vi "Errors to Item Names.vi"(5 "scope":T1, 7 "error list <top>":variant, 8 "error in (no error)":errorcluster, 11 "displayed errors in":T2[](array[typedef])) -> (0 "error out":errorcluster, 2 "item names":string[][](array[string]), 3 "displayed errors out":T2[](array[typedef]))   [LabVIEW 2017]
uses:
  Error List/Error Owner and ID.ctl
  Error List/Scope.ctl
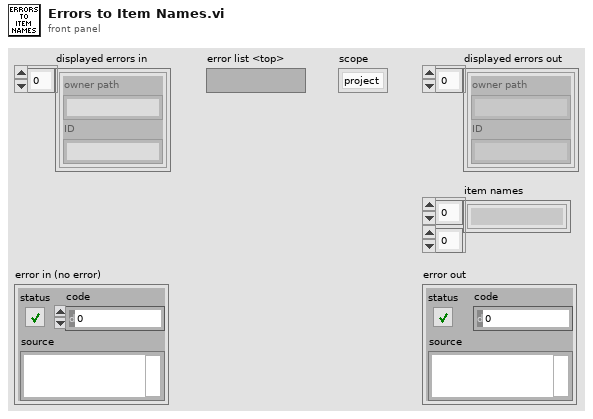
[diagram p1: front panel]
types:
  T1 = typedef "Scope.ctl" = enum16{"project", "global"}
  T2 = typedef "Error Owner and ID.ctl" = cluster{"owner path":string, "ID":string}
  T3 = typedef "Error Owners and IDs.ctl" = cluster{"owner path":string, "error IDs":string[]}
  T4 = typedef "Error File Management.lvlib/NI Error.ctl" = errorcluster
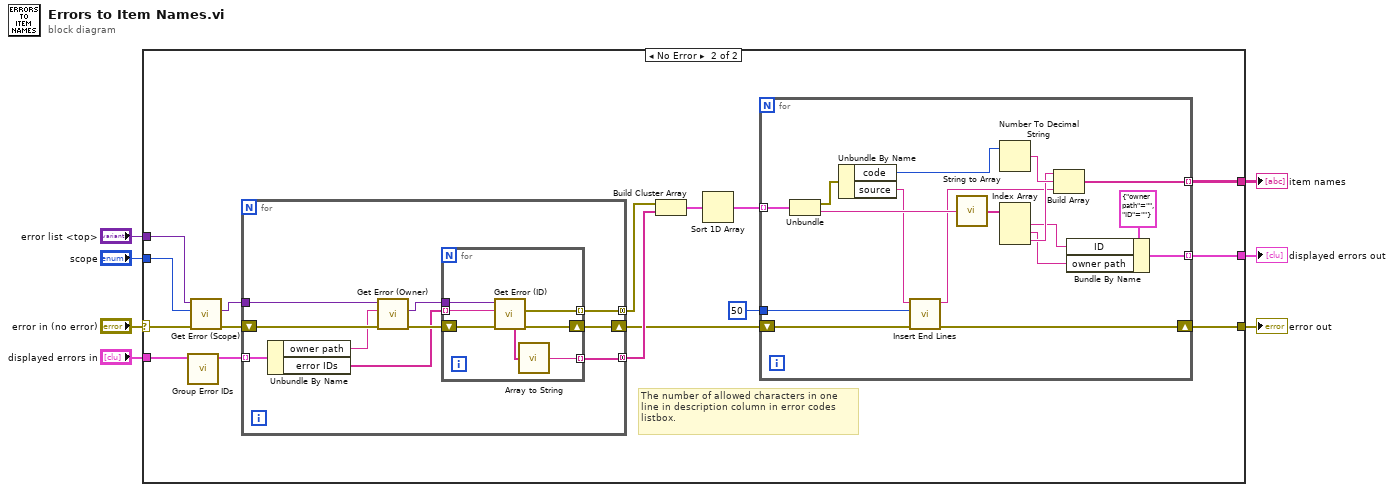
[diagram p0: block diagram]
diagram:
  n1 = case shown="No Error" "error in (no error)" {
    selector: "error in (no error)" -> [w9 w19]
    tunnel: "displayed errors in" -> [w8 w14]
    tunnel: [w9 w11] -> w5
    tunnel: [w8 w15] -> w4
    tunnel: "error list <top>" -> [_ w18]
    tunnel: "scope" -> [_ w17]
    tunnel: [_ w16] -> w1
    frame Error {
    }
    frame No Error {
      # "The number of allowed characters in one line in description column in error codes listbox."
      n2 = call "Group Error IDs.vi"("error IDs in"=w14) -> ("grouped error IDs"=w13:T3[])  [unwired: 9 in, 1 out]
      n3 = call "Get Error (Scope).vi"("error in (no error)"=w19, "scope"=w17, "error list <top>"=w18) -> ("error out"=w25:errorcluster, "error list <scope>"=w24:variant)  [unwired: 5 in, 2 out]
      n4 = for {
        shift-right: [w32] -> w12
        shift-left: w25 -> [w35]
        tunnel: w24 -> [w34]
        tunnel: [w30] -> w23 mode=concatenating
        tunnel: w13 -> [w29] mode=indexing
        tunnel: [w26] -> w22 mode=concatenating
        n5 = Unbundle By Name(w29) -> ("owner path"=w28:string, "error IDs"=w27:string[])
        n6 = call "Get Error (Owner).vi"("error in (no error)"=w35, "owner"=w28, "error list <scope>"=w34) -> ("error out"=w33:errorcluster, "error list <owner>"=w31:variant)  [unwired: 5 in, 2 out]
        n7 = for {
          shift-right: [w41] -> w32
          shift-left: w33 -> [w42]
          tunnel: w27 -> [w39] mode=indexing
          tunnel: [w38] -> w30 mode=indexing
          tunnel: w31 -> [w40]
          tunnel: [w37] -> w26 mode=indexing
          n8 = call "Get Error (ID).vi"("error in (no error)"=w42, "ID"=w39, "error list <owner>"=w40) -> ("error out"=w41:errorcluster, "error"=w38:T4, "attributes"=w36:string[])  [unwired: 4 in, 2 out]
          n9 = call "Array to String.vi"("array"=w36) -> ("string"=w37:string)  [unwired: 1 in]
        }
      }
      n10 = Build Cluster Array(w23, w22) -> (w20:cluster{"error":T4, "string":string}[])
      n11 = Sort 1D Array(array=w20) -> (sorted array=w21:cluster{"error":T4, "string":string}[])
      n12 = for {
        tunnel: w21 -> [w59] mode=indexing
        tunnel: [w53] -> w16 mode=indexing
        tunnel: [w48] -> w15 mode=indexing
        shift-right: [w44] -> w11
        shift-left: w12 -> [w47]
        tunnel: 50 ("max chars in line") -> [w43]
        n13 = Unbundle(w59) -> ("error"=w57:T4, "string"=w58:string)
        n14 = Unbundle By Name(w57) -> ("code"=w56:i32, "source"=w46:string)
        n15 = call "Insert End Lines.vi"("error in (no error)"=w47, "max chars in line"=w43, "string in"=w46) -> ("error out"=w44:errorcluster, "string with end lines"=w45:string)  [unwired: 7 in]
        n16 = call "String to Array.vi"("string"=w58) -> ("array"=w55:string[])  [unwired: 1 in]
        n17 = Number To Decimal String(number=w56) -> (decimal integer string=w54:string)  [unwired: 1 in]
        n18 = Index Array(array=w55) -> (element #1=w50:string, element #2=w49:string, element #3=w52:string)  [unwired: 3 in]
        n19 = Build Array(w52, w54, w45) -> (w53:string[])
        n20 = Bundle By Name(cluster=T2 {"owner path"="", "ID"=""} ("owner error"), "ID"=w50, "owner path"=w49) -> (w48:T2)
      }
    }
  }
  "error out" <- w5
  "displayed errors out" <- w4
  "item names" <- w1
